vi "Stop Msg.vi"(6 "Priority Message? (F)":bool, 8 "error in (no error)":errorcluster, 11 "Queue in":refnum<queue>) -> (0 "error out":errorcluster)   [LabVIEW 2018, in "Acquisition.lvlib"]
uses:
  Acquisition.lvlib
  Support/Message Queue/Message Cluster.ctl
  Support/Message Queue/Enqueue Message (Single).vi
  support/Message Queue/Message Queue.lvlib
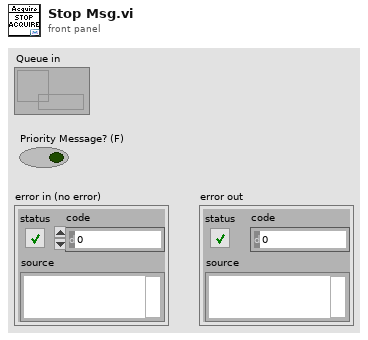
[diagram p1: front panel]
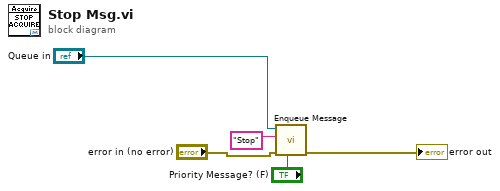
[diagram p0: block diagram]
diagram:
  n1 = call-poly "Enqueue Message.vi"("Priority Message? (F)"="Priority Message? (F)", "error in (no error)"="error in (no error)", "Message"="Stop", "Message Queue"="Queue in") -> ("error out"=→"error out":errorcluster)  [unwired: 6 in, 1 out]
